vi "CSM - Check Mapping Relationship in Broadcast Registry.vi"(8 "error in (no error)":errorcluster, 10 "CSM Name":string, 11 "Broadcast Name":string) -> (0 "error out":errorcluster, 3 "Mapping Relationships":T2(array[cluster]))   [LabVIEW 2017, in "Communicable State Machine.lvlib"]
doc: "Checks all registration relationships corresponding to a specific broadcast name of a CSM module.\n\n\n> [!NOTE] <b>CSM Broadcast</b>\n>\n> Broadcasts in CSM are divided into three types: Status Broadcast, Interrupt Broadcast, and State Broadcast. The module pushes the Status Broadcast to all modules registered to that Status Broadcast. Status Broadcast and Interrupt Broadcast are explicitly called broadcasts, while State Broadcast is an implicit broadcast. When a subscription relationship exists, the State Broadcast is automatically triggered when the CSM completes a certain state.\n>\n> - <b>Status Broadcast</b>: Normal priority broadcast. Similar to asynchronous messages, it is passed via the low-priority queue. It is processed sequentially when other unprocessed asynchronous messages or Status Broadcasts exist in the module.\n> - <b>Interrupt Broadcast</b>: High priority broadcast. Similar to synchronous messages, it is passed via the high-priority queue. It is processed first when other low-priority asynchronous messages or Status Broadcasts exist in the module. However, if other unprocessed synchronous messages or Interrupt Broadcasts exist, it is processed sequentially.\n> - <b>State Broadcast</b>: State Broadcast is an implicit broadcast. When a subscription relationship exists, the State Broadcast is automatically triggered when the CSM completes a certain state. The argument for the State Broadcast is the Response of the CSM state.\n\n\n> [!NOTE] <b>CSM Registration</b>\n>\n> Registration associates a broadcast with a bound interface (API). When the broadcast is triggered, the bound interface (API) is called. Registrations can also be cancelled. In CSM, there are two types of broadcasts:\n>\n> 1. <b>Broadcast</b>: Broadcast explicitly called by the module sending the broadcast message. Arguments need to be explicitly provided.\n> 2. <b>State</b>: Any state of a CSM module can also be registered to. The argument received by the triggered API is the Response of the CSM state.\n>\n> // Register `[Broadcast Message Name]@[SourceModule] >> [Bound API]@[TargetModule] -><register> // [Comments]`// Unregister `[Broadcast Message Name]@[SourceModule] >> [Bound API]@[TargetModule] -><unregister> // [Comments]`\n\n> - <b>Broadcast Message Name</b>: Defined by the source module. Refer to \"CSM Broadcast Format Parsing\" for details.\n> - <b>Source Module</b>: The broadcasting module. If subscribing to broadcasts from any module, the source module can be represented by `*`.\n> - <b>Bound API</b>: Defined by the target module. It is the external interface of the target module.\n> - <b>Target Module</b>: The module where the bound API resides. When indicating registration to the current module within a CSM module, it can be ignored. The preceding `@` separator is also omitted.\n> - `<register>` / `<unregister>`: Definition of the Register/Unregister operation type.\n> - <b>Comments</b>: Comment information, which will not be parsed.\n\n\n-- <b>Controls</b> --\n- <b>CSM Name</b>: CSM module name.\n- <b>Broadcast Name</b>: Name of the broadcast.\n\n-- <b>Indicators</b> --\n- <b>Mapping Relationships</b>: All registration relationships corresponding to the specific broadcast name of the current CSM module."
uses:
  Communicable State Machine.lvlib
  CSM - Broadcast Message Type.ctl
  _Support/ChangeFlag/FlagInstance-CSMQ FGV.vi
  _Support/ChangeFlag/FlagInstance-Broadcast Cache.vi
  _Support/ChangeFlag/ChangeFlag-Read.vi
  _Support/FGV-BroadcastRegistry/FGV-BroadcastRegistry(lvlibp).vi
  CSM - List Modules.vi
  _Support/BroadcastRegistry/HelperVI/Broadcast Item Key.vi
  _Shared/Trim Single-line Text.vi
  _Support/ChangeFlag/ChangeFlagDB.vi
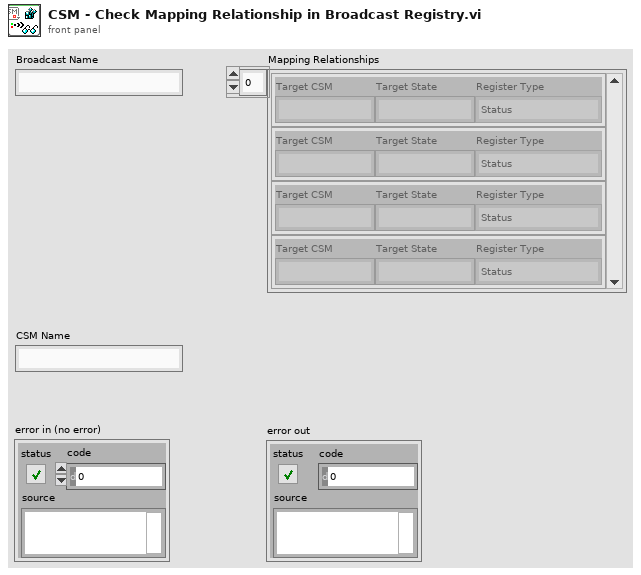
[diagram p1: front panel]
types:
  T1 = typedef "Communicable State Machine.lvlib/CSM - Broadcast Message Type.ctl" = enum16{"<Null>", "Status", "Interrupt"}
  T2 = cluster{"Target CSM":string, "Target State":string, "Register Type":T1}[]
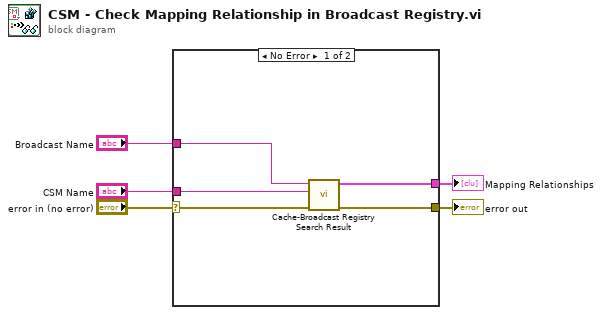
[diagram p0: block diagram]
diagram:
  n1 = case shown="No Error" "error in (no error)" {
    selector: "error in (no error)" -> [w7 w11]
    tunnel: "Broadcast Name" -> [w10 _]
    tunnel: "CSM Name" -> [w9 _]
    tunnel: [w8 _] -> w3
    tunnel: [w6 w11] -> w1
    frame No Error {
      n2 = call "Cache-Broadcast Registry Search Result.vi"("error in (no error)"=w7, "CSM Name"=w9, "Broadcast State"=w10) -> ("error out"=w6:errorcluster, "Array"=w8:T2)  [unwired: 7 in]
    }
    frame Error {
    }
  }
  "Mapping Relationships" <- w3
  "error out" <- w1
